vi "OutToExcel.vi"(9 "Table Control":string[][](table), 10 "Running":string[][](table), 11 "Report Template":path=path "c:/m100/data/AT.xls") -> ()   [LabVIEW 2012]
uses:
  <vilib>/Utility/NIReport.llb/NI_report.lvclass
  <vilib>/Utility/NIReport.llb/Append Text Table to Report (wrap).vi
  Global1.vi
  <vilib>/Utility/NIReport.llb/Excel/NI_Excel.lvclass
  <vilib>/addons/_office/NI_ReportGenerationToolkit.lvlib
panel:
  out "error out 2":errorcluster
  out "Row Headers 2":string[](array[string])
  out "Row Headers":string[](array[string])
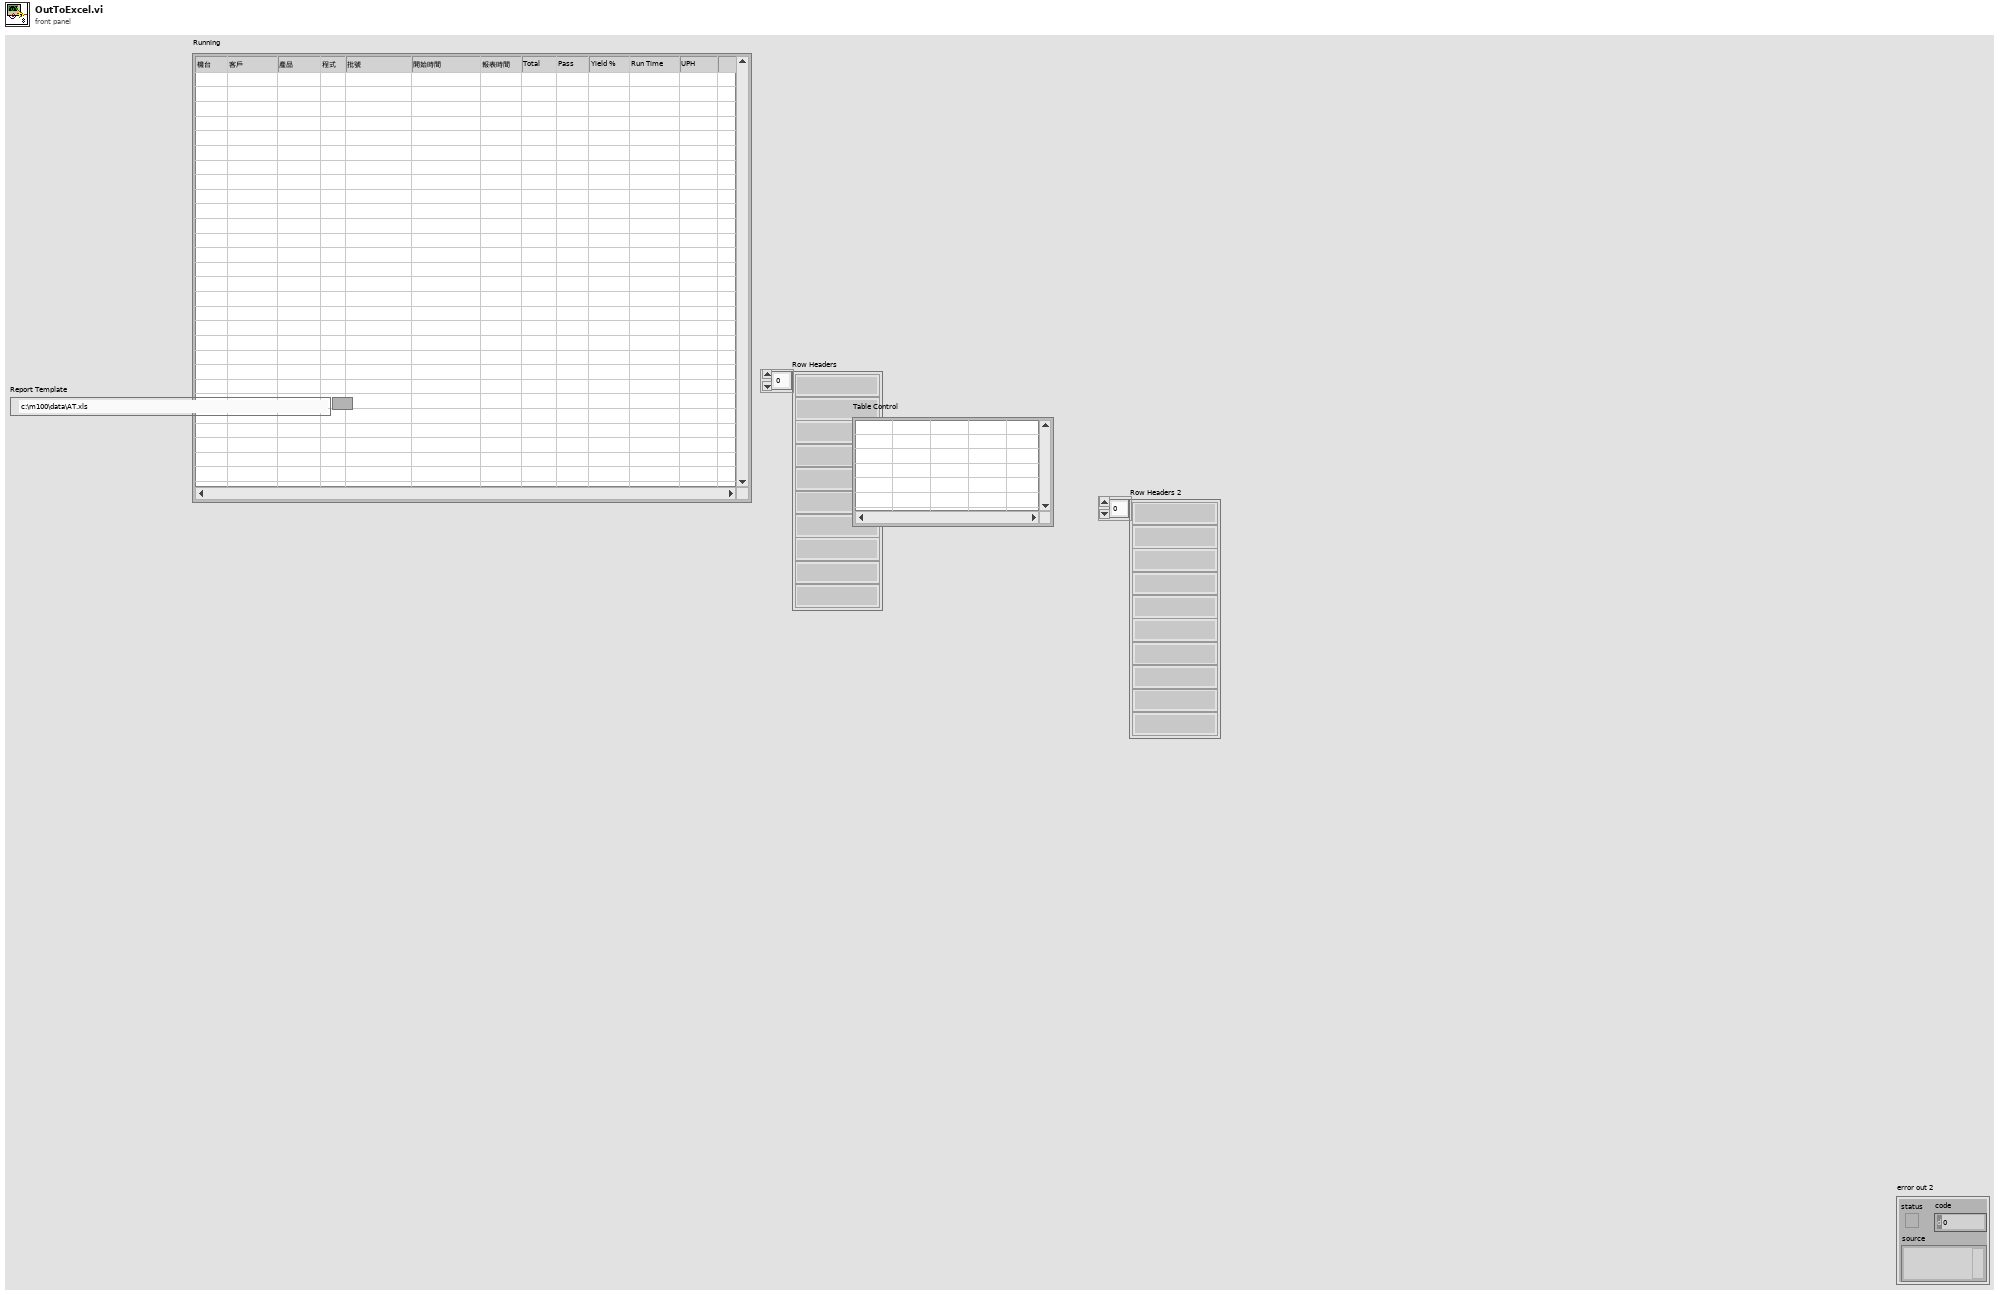
[diagram p1: front panel]
types:
  T1 = enum16{"Standard Report", "HTML", "Word", "Excel"}
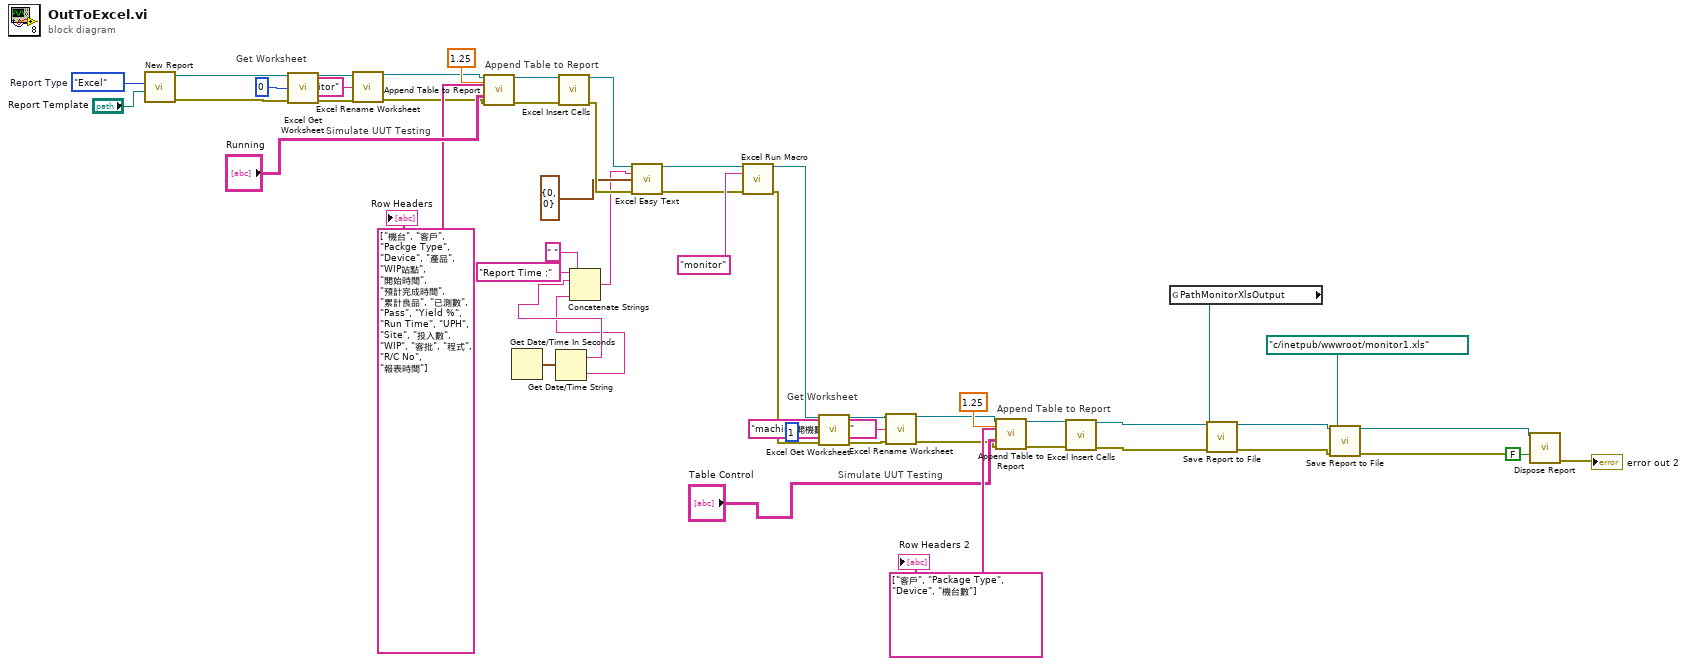
[diagram p0: block diagram]
diagram:
  w38 = string[] ["客戶", "Package Type", "Device", "機台數"] ("row headers")
  w46 = string[] ["機台", "客戶", "Packge Type", "Device", "產品", "WIP站點", "開始時間", "預計完成時間", "累計良品", "已測數", "Pass", "Yield %", "Run Time", "UPH", "Site", "投入數", "WIP", "客批", "程式", "R/C No", "報表時間"] ("row headers")
  w50 = T1."Excel"  # Report Type
  # "Simulate UUT Testing"
  # "Append Table to Report"
  # "Get Worksheet"
  # "Simulate UUT Testing"
  # "Append Table to Report"
  # "Get Worksheet"
  n1 = call <vilib>:"New Report.vi"("report type"=w50, "template (empty)"="Report Template") -> ("report out"=w43:refnum<class "NI_report.lvclass">, "error out"=w42:errorcluster)  [unwired: 12 in]
  n2 = call <vilib>:"Excel Get Worksheet.vi"("report in"=w43, "worksheet index (0)"=0, "error in (no error)"=w42) -> ("report out"=w31:refnum<class "NI_report.lvclass">, "error out"=w29:errorcluster)  [unwired: 11 in]
  n3 = call <vilib>:"Excel Rename Worksheet.vi"("report in"=w31, "worksheet name (\"\")"="monitor" ("worksheet name (\"\")"), "error in (no error)"=w29) -> ("report out"=w30:refnum<class "NI_report.lvclass">, "error out"=w28:errorcluster)  [unwired: 11 in]
  n4 = call-poly <vilib>:"Append Table to Report.vi"("report in"=w30, "column width (1)"=1.25, "column headers"=w46, "text data"="Running", "error in (no error)"=w28) -> ("report out"=w45:refnum<class "NI_report.lvclass">, "error out"=w44:errorcluster)  [unwired: 7 in, 2 out]
  n5 = Get Date/Time In Seconds() -> (seconds since 1Jan1904=w10:timestamp)
  n6 = Get Date/Time String(seconds (now)=w10) -> (date string=w9:string, time string=w7:string)  [unwired: 2 in]
  n7 = call <vilib>:"Excel Insert Cells.vi"("report in"=w45, "error in (no error)"=w44) -> ("report out"=w14:refnum<class "NI_report.lvclass">, "error out"=w13:errorcluster)  [unwired: 12 in]
  n8 = Concatenate Strings("Report Time :" ("string"), w9, " " ("string"), w7) -> (w6:string)
  n9 = call <vilib>:"Excel Easy Text.vi"("report in"=w14, "text"=w6, "start (-1, -1)"=cluster{"row":i32, "column":i32} {"row"=0, "column"=0} ("end (-1, -1)"), "error in (no error)"=w13) -> ("report out"=w16:refnum<class "NI_report.lvclass">, "error out"=w15:errorcluster)  [unwired: 7 in, 3 out]
  n10 = call <vilib>:"Excel Run Macro.vi"("report in"=w16, "macro name"="monitor", "error in (no error)"=w15) -> ("report out"=w33:refnum<class "NI_report.lvclass">, "error out"=w32:errorcluster)  [unwired: 10 in, 1 out]
  n11 = call <vilib>:"Excel Get Worksheet.vi"("report in"=w33, "worksheet index (0)"=1, "error in (no error)"=w32) -> ("report out"=w26:refnum<class "NI_report.lvclass">, "error out"=w24:errorcluster)  [unwired: 11 in]
  n12 = call <vilib>:"Excel Rename Worksheet.vi"("report in"=w26, "worksheet name (\"\")"="machine開機數及分布" ("worksheet name (\"\")"), "error in (no error)"=w24) -> ("report out"=w25:refnum<class "NI_report.lvclass">, "error out"=w23:errorcluster)  [unwired: 11 in]
  n13 = call-poly <vilib>:"Append Table to Report.vi"("report in"=w25, "column width (1)"=1.25, "column headers"=w38, "text data"="Table Control", "error in (no error)"=w23) -> ("report out"=w37:refnum<class "NI_report.lvclass">, "error out"=w36:errorcluster)  [unwired: 7 in, 2 out]
  n14 = call <vilib>:"Excel Insert Cells.vi"("report in"=w37, "error in (no error)"=w36) -> ("report out"=w20:refnum<class "NI_report.lvclass">, "error out"=w21:errorcluster)  [unwired: 12 in]
  n15 = global read "Global1.vi" "PathMonitorXlsOutput"() -> (w19:path)
  n16 = call-dynamic "Save Report to File.vi"("report in"=w20, "report file path"=w19, "error in (no error)"=w21) -> ("report out"=w5:refnum<class "NI_report.lvclass">, "error out"=w4:errorcluster)  [unwired: 11 in]
  n17 = call-dynamic "Save Report to File.vi"("report in"=w5, "report file path"=path "c:/inetpub/wwwroot/monitor1.xls", "error in (no error)"=w4) -> ("report out"=w3:refnum<class "NI_report.lvclass">, "error out"=w2:errorcluster)  [unwired: 11 in]
  n18 = call-dynamic "Dispose Report.vi"("report in"=w3, "save changes? (F)"=FALSE, "error in (no error)"=w2) -> ("error out"=→"error out 2":errorcluster)  [unwired: 12 in]
  "Row Headers" <- w46
  "Row Headers 2" <- w38
